vi "欧姆龙PLC通讯Fans UDP-解码读出来数据.vi"(8 "解码类型":T3, 9 "16bit寄存器个数":u16=2, 10 "从PLC读取信息 in":T1 {"Mark拍照点坐标"."X" format="%#.3f"}, 11 "PLCoutput":string) -> (0 "解码成触发信号":bool[](array[boolean]), 1 "Mark点坐标4个":T2[](array[typedef]) {"X" format="%#.3f"}, 2 "从PLC读取信息 out":T1 {"Mark拍照点坐标"."X" format="%#.3f"}, 3 "回传数据长度大于0":bool, 5 "解码成U16数组":u16[](array[numeric]))   [LabVIEW 2014]
uses:
  Controls/XYPos.ctl
panel:
  out "数字":i32
  out "2":u32
  out "1":u32
  out "3":u32
  out "4":u32
  out "5":u32
  in  "data  解码后是-998777":string
  out "I32数组":i32[](array[numeric])
  out "U32数组":u32[](array[numeric])
  in  "data 数值16进制7530=30000":string
  in  "data 数值16进制54=84":string
  out "解码成I16数组":i16[](array[numeric])
  out "无符号字节数组":u8[](array[numeric])
  out "子字符串":string
  # "传输时，低位在前高位在后20000    20001"
  # "C287   FFF0"
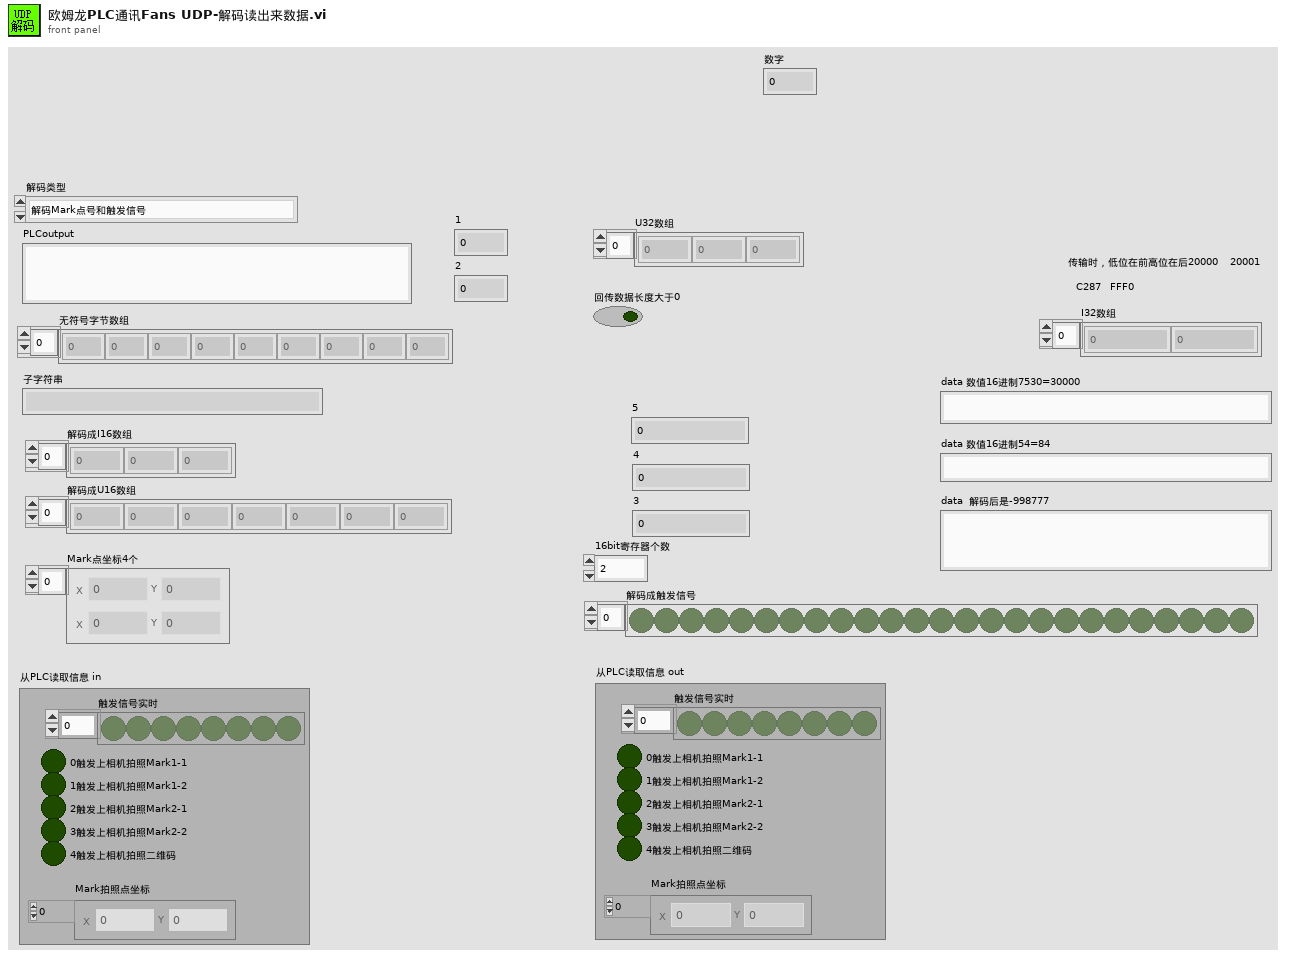
[diagram p1: front panel]
types:
  T1 = typedef "控件-UDP从PLC读取信息.ctl" = cluster{"触发信号实时":bool[], "0触发上相机拍照Mark1-1":bool, "1触发上相机拍照Mark1-2":bool, "2触发上相机拍照Mark2-1":bool, "3触发上相机拍照Mark2-2":bool, "4触发上相机拍照二维码":bool, "Mark拍照点坐标":T2[]}
  T2 = typedef "XYPos.ctl" = cluster{"X":dbl, "Y":dbl}
  T3 = typedef "控件-UDP解码类型.ctl" = enum16{"解码Mark点号和触发信号", "解码Mark点坐标"}
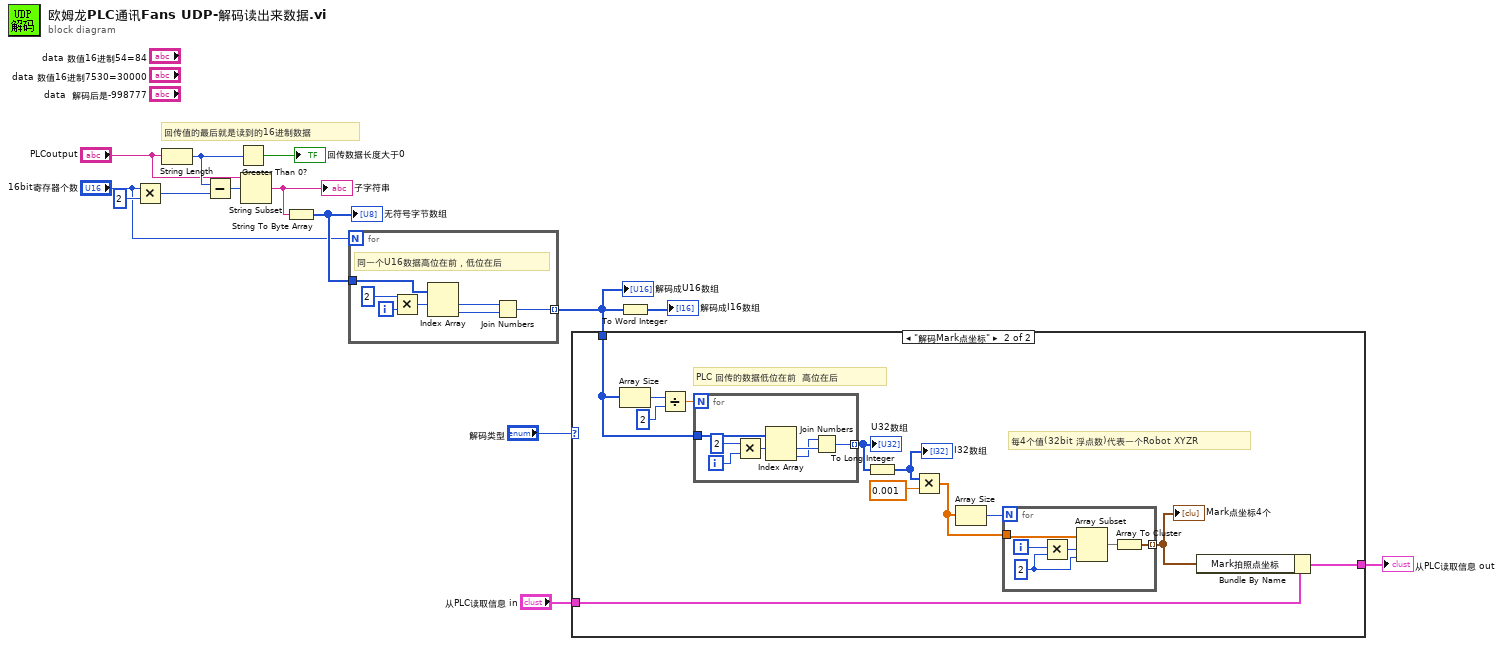
[diagram p0: block diagram]
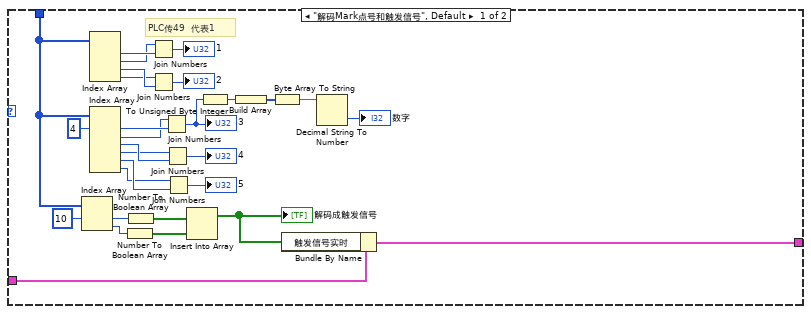
[diagram p2: hidden frame]
diagram:
  # "回传值的最后就是读到的16进制数据"
  n1 = Multiply(x="16bit寄存器个数", y=u16 2) -> (x*y=w10:u16)
  n2 = String Length(string="PLCoutput") -> (length=w13:i32)
  n3 = Subtract(x=w13, y=w10) -> (x-y=w12:i32)
  n4 = Greater Than 0?(x=w13) -> (x > 0?=→"回传数据长度大于0":bool)
  n5 = String Subset(string="PLCoutput", offset (0)=w12) -> (substring=w8:string)  [unwired: 1 in]
  "子字符串" <- w8
  n6 = String To Byte Array(string=w8) -> (unsigned byte array=w9:u8[])
  "无符号字节数组" <- w9
  n7 = for {
    N: "16bit寄存器个数" -> [_]
    tunnel: w9 -> [w21]
    tunnel: [w17] -> w3 mode=indexing
    i -> [w20]
    # "同一个U16数据高位在前，低位在后"
    n8 = Multiply(x=2, y=w20) -> (x*y=w18:i32)
    n9 = Index Array(array=w21, index #1=w18) -> (element #1=w16:u8, element #2=w15:u8)  [unwired: 1 in]
    n10 = Join Numbers(hi=w16, lo=w15) -> ((hi.lo)=w17:u16)
  }
  "解码成U16数组" <- w3
  n11 = case shown="\"解码Mark点坐标\"" "解码类型" {
    tunnel: w3 -> [w34 w59]
    tunnel: "从PLC读取信息 in" -> [w29 w53]
    tunnel: [w28 w51] -> w1
    frame "解码Mark点号和触发信号", Default {
      # "PLC传49  代表1"
      n12 = Index Array(array=w34, index #1=10 ("索引")) -> (element #1=w50:u16, element #2=w49:u16)  [unwired: 1 in]
      n13 = Index Array(array=w34) -> (element #1=w33:u16, element #2=w32:u16, element #3=w31:u16, element #4=w30:u16)  [unwired: 4 in]
      n14 = Index Array(array=w34, index #1=4 ("索引")) -> (element #1=w45:u16, element #2=w44:u16, element #3=w43:u16, element #4=w42:u16, element #5=w41:u16, element #6=w40:u16)  [unwired: 5 in]
      n15 = Number To Boolean Array(number=w49) -> (Boolean array=w47:bool[])
      n16 = Number To Boolean Array(number=w50) -> (Boolean array=w48:bool[])
      n17 = Join Numbers(hi=w32, lo=w33) -> ((hi.lo)=→"1":u32)
      n18 = Join Numbers(hi=w30, lo=w31) -> ((hi.lo)=→"2":u32)
      n19 = Join Numbers(hi=w44, lo=w45) -> ((hi.lo)=w37:u32)
      "3" <- w37
      n20 = Join Numbers(hi=w42, lo=w43) -> ((hi.lo)=→"4":u32)
      n21 = Join Numbers(hi=w40, lo=w41) -> ((hi.lo)=→"5":u32)
      n22 = Insert Into Array(array=w48, new element=w47) -> (w27:bool[])  [unwired: 1 in]
      "解码成触发信号" <- w27
      n23 = To Unsigned Byte Integer(number=w37) -> (unsigned 8bit integer=w38:u8)
      n24 = Build Array(w38) -> (w39:u8[])
      n25 = Byte Array To String(unsigned byte array=w39) -> (string=w36:string)
      n26 = Bundle By Name(cluster=w29, "触发信号实时"=w27) -> (w28:T1)
      n27 = Decimal String To Number(string=w36) -> (number=→"数字":i32)  [unwired: 2 in, 1 out]
    }
    frame "解码Mark点坐标" {
      # "每4个值(32bit 浮点数)代表一个Robot XYZR"
      # "PLC 回传的数据低位在前  高位在后"
      n28 = Array Size(array=w59) -> (size(s)=w62:i32)
      n29 = Divide(x=w62, y=2) -> (x/y=w60:dbl)
      n30 = for {
        N: w60 -> [_]
        tunnel: w59 -> [w71]
        tunnel: [w73] -> w58 mode=indexing
        i -> [w75]
        n31 = Multiply(x=2, y=w75) -> (x*y=w72:i32)
        n32 = Index Array(array=w71, index #1=w72) -> (element #1=w70:u16, element #2=w69:u16)  [unwired: 1 in]
        n33 = Join Numbers(hi=w69, lo=w70) -> ((hi.lo)=w73:u32)
      }
      "U32数组" <- w58
      n34 = To Long Integer(number=w58) -> (32bit integer=w57:i32[])
      "I32数组" <- w57
      n35 = Multiply(x=w57, y=0.001) -> (x*y=w54:dbl[])
      n36 = Array Size(array=w54) -> (size(s)=w55:i32)
      n37 = for {
        N: w55 -> [_]
        tunnel: w54 -> [w67]
        tunnel: [w63] -> w52 mode=indexing
        i -> [w65]
        w64 = 2 ("长度")
        n38 = Multiply(x=w65, y=w64) -> (x*y=w66:i32)
        n39 = Array Subset(array=w67, index=w66, length=w64) -> (w68:dbl[])
        n40 = Array To Cluster(array=w68) -> (cluster=w63:cluster{"[0]":dbl, "[1]":dbl})
      }
      "Mark点坐标4个" <- w52
      n41 = Bundle By Name(cluster=w53, "Mark拍照点坐标"=w52) -> (w51:T1)
    }
  }
  "从PLC读取信息 out" <- w1
  n42 = To Word Integer(number=w3) -> (16bit integer=→"解码成I16数组":i16[])
